vi "Lift.vi"   [LabVIEW 2017]
uses:
  <userlib>/836-Library/System/QCP_V2/QCPSupportCode/QCPData.ctl
  <userlib>/836-Library/System/QCP_V2/QCPSupportCode/QCP_GetDbl.vi
types:
  T1 = typedef "Semaphore RefNum" = refnum<k1>
  T2 = cluster{"Data Value Refnum":refnum<data-value>, "semaphore":T1}
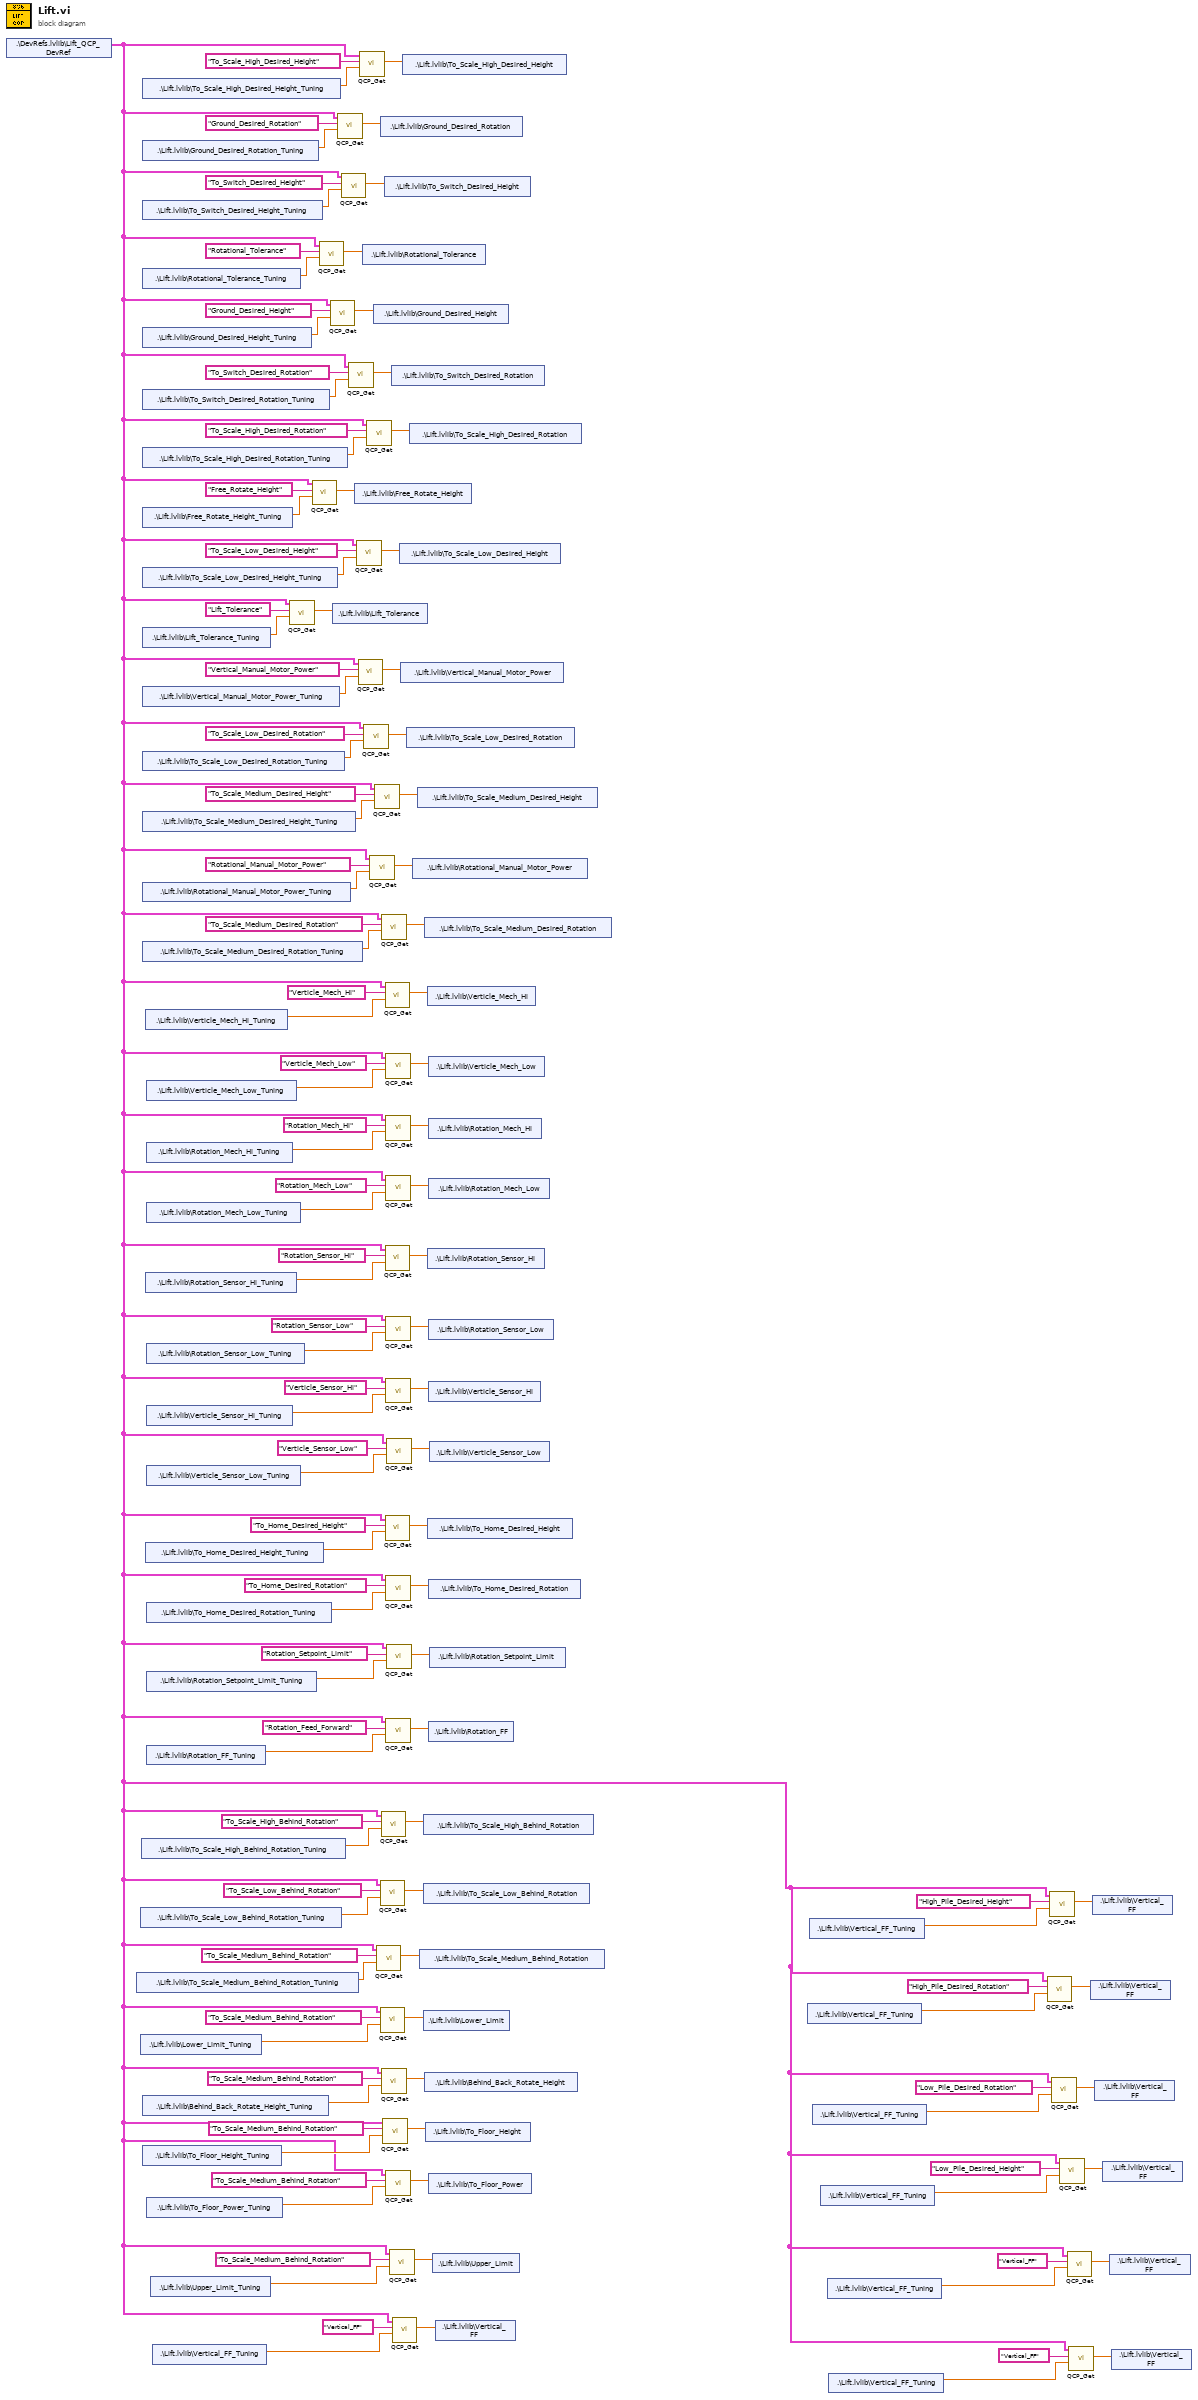
[diagram p0: block diagram]
diagram:
  n1 = shared-variable ".\\DevRefs.lvlib\\Lift_QCP_DevRef"() -> (w1:T2)  [unwired: 1 in, 1 out]
  n2 = shared-variable ".\\Lift.lvlib\\To_Scale_Medium_Behind_Rotation_Tuninig"() -> (w38:dbl)  [unwired: 1 in, 1 out]
  n3 = shared-variable ".\\Lift.lvlib\\To_Scale_Low_Behind_Rotation_Tuning"() -> (w43:dbl)  [unwired: 1 in, 1 out]
  n4 = shared-variable ".\\Lift.lvlib\\Lower_Limit_Tuning"() -> (w37:dbl)  [unwired: 1 in, 1 out]
  n5 = shared-variable ".\\Lift.lvlib\\To_Scale_High_Behind_Rotation_Tuning"() -> (w44:dbl)  [unwired: 1 in, 1 out]
  n6 = shared-variable ".\\Lift.lvlib\\To_Scale_High_Desired_Height_Tuning"() -> (w91:dbl)  [unwired: 1 in, 1 out]
  n7 = shared-variable ".\\Lift.lvlib\\Ground_Desired_Rotation_Tuning"() -> (w95:dbl)  [unwired: 1 in, 1 out]
  n8 = shared-variable ".\\Lift.lvlib\\To_Switch_Desired_Height_Tuning"() -> (w85:dbl)  [unwired: 1 in, 1 out]
  n9 = shared-variable ".\\Lift.lvlib\\Rotational_Tolerance_Tuning"() -> (w92:dbl)  [unwired: 1 in, 1 out]
  n10 = shared-variable ".\\Lift.lvlib\\Ground_Desired_Height_Tuning"() -> (w96:dbl)  [unwired: 1 in, 1 out]
  n11 = shared-variable ".\\Lift.lvlib\\To_Switch_Desired_Rotation_Tuning"() -> (w84:dbl)  [unwired: 1 in, 1 out]
  n12 = shared-variable ".\\Lift.lvlib\\To_Scale_High_Desired_Rotation_Tuning"() -> (w90:dbl)  [unwired: 1 in, 1 out]
  n13 = shared-variable ".\\Lift.lvlib\\Free_Rotate_Height_Tuning"() -> (w97:dbl)  [unwired: 1 in, 1 out]
  n14 = shared-variable ".\\Lift.lvlib\\To_Scale_Low_Desired_Height_Tuning"() -> (w89:dbl)  [unwired: 1 in, 1 out]
  n15 = shared-variable ".\\Lift.lvlib\\Lift_Tolerance_Tuning"() -> (w94:dbl)  [unwired: 1 in, 1 out]
  n16 = shared-variable ".\\Lift.lvlib\\Vertical_Manual_Motor_Power_Tuning"() -> (w83:dbl)  [unwired: 1 in, 1 out]
  n17 = shared-variable ".\\Lift.lvlib\\To_Scale_Low_Desired_Rotation_Tuning"() -> (w88:dbl)  [unwired: 1 in, 1 out]
  n18 = shared-variable ".\\Lift.lvlib\\To_Scale_Medium_Desired_Height_Tuning"() -> (w87:dbl)  [unwired: 1 in, 1 out]
  n19 = shared-variable ".\\Lift.lvlib\\Rotational_Manual_Motor_Power_Tuning"() -> (w93:dbl)  [unwired: 1 in, 1 out]
  n20 = shared-variable ".\\Lift.lvlib\\To_Scale_Medium_Desired_Rotation_Tuning"() -> (w86:dbl)  [unwired: 1 in, 1 out]
  n21 = shared-variable ".\\Lift.lvlib\\Behind_Back_Rotate_Height_Tuning"() -> (w32:dbl)  [unwired: 1 in, 1 out]
  n22 = shared-variable ".\\Lift.lvlib\\To_Floor_Height_Tuning"() -> (w31:dbl)  [unwired: 1 in, 1 out]
  n23 = shared-variable ".\\Lift.lvlib\\Verticle_Mech_Hi_Tuning"() -> (w82:dbl)  [unwired: 1 in, 1 out]
  n24 = shared-variable ".\\Lift.lvlib\\Rotation_Sensor_Hi_Tuning"() -> (w59:dbl)  [unwired: 1 in, 1 out]
  n25 = shared-variable ".\\Lift.lvlib\\To_Home_Desired_Height_Tuning"() -> (w58:dbl)  [unwired: 1 in, 1 out]
  n26 = shared-variable ".\\Lift.lvlib\\Verticle_Mech_Low_Tuning"() -> (w77:dbl)  [unwired: 1 in, 1 out]
  n27 = shared-variable ".\\Lift.lvlib\\Rotation_Mech_Hi_Tuning"() -> (w76:dbl)  [unwired: 1 in, 1 out]
  n28 = shared-variable ".\\Lift.lvlib\\Rotation_Mech_Low_Tuning"() -> (w71:dbl)  [unwired: 1 in, 1 out]
  n29 = shared-variable ".\\Lift.lvlib\\Rotation_Sensor_Low_Tuning"() -> (w64:dbl)  [unwired: 1 in, 1 out]
  n30 = shared-variable ".\\Lift.lvlib\\Verticle_Sensor_Hi_Tuning"() -> (w65:dbl)  [unwired: 1 in, 1 out]
  n31 = shared-variable ".\\Lift.lvlib\\To_Home_Desired_Rotation_Tuning"() -> (w53:dbl)  [unwired: 1 in, 1 out]
  n32 = shared-variable ".\\Lift.lvlib\\Rotation_FF_Tuning"() -> (w49:dbl)  [unwired: 1 in, 1 out]
  n33 = shared-variable ".\\Lift.lvlib\\To_Floor_Power_Tuning"() -> (w26:dbl)  [unwired: 1 in, 1 out]
  n34 = shared-variable ".\\Lift.lvlib\\Verticle_Sensor_Low_Tuning"() -> (w70:dbl)  [unwired: 1 in, 1 out]
  n35 = shared-variable ".\\Lift.lvlib\\Rotation_Setpoint_Limit_Tuning"() -> (w50:dbl)  [unwired: 1 in, 1 out]
  n36 = shared-variable ".\\Lift.lvlib\\Upper_Limit_Tuning"() -> (w25:dbl)  [unwired: 1 in, 1 out]
  n37 = shared-variable ".\\Lift.lvlib\\Vertical_FF_Tuning"() -> (w20:dbl)  [unwired: 1 in, 1 out]
  n38 = call-poly <userlib>:"QCP_Get.vi"("Tuning Value"=w94, "Value Name"="Lift_Tolerance", "QCP_DevRef_In"=w1) -> ("Value"=w109:dbl)  [unwired: 6 in, 2 out]
  n39 = call-poly <userlib>:"QCP_Get.vi"("Tuning Value"=w97, "Value Name"="Free_Rotate_Height", "QCP_DevRef_In"=w1) -> ("Value"=w112:dbl)  [unwired: 6 in, 2 out]
  n40 = call-poly <userlib>:"QCP_Get.vi"("Tuning Value"=w92, "Value Name"="Rotational_Tolerance", "QCP_DevRef_In"=w1) -> ("Value"=w104:dbl)  [unwired: 6 in, 2 out]
  n41 = call-poly <userlib>:"QCP_Get.vi"("Tuning Value"=w96, "Value Name"="Ground_Desired_Height", "QCP_DevRef_In"=w1) -> ("Value"=w111:dbl)  [unwired: 6 in, 2 out]
  n42 = shared-variable ".\\Lift.lvlib\\Lift_Tolerance"(w109) -> ()  [unwired: 1 in, 1 out]
  n43 = call-poly <userlib>:"QCP_Get.vi"("Tuning Value"=w95, "Value Name"="Ground_Desired_Rotation", "QCP_DevRef_In"=w1) -> ("Value"=w110:dbl)  [unwired: 6 in, 2 out]
  n44 = call-poly <userlib>:"QCP_Get.vi"("Tuning Value"=w85, "Value Name"="To_Switch_Desired_Height", "QCP_DevRef_In"=w1) -> ("Value"=w100:dbl)  [unwired: 6 in, 2 out]
  n45 = call-poly <userlib>:"QCP_Get.vi"("Tuning Value"=w84, "Value Name"="To_Switch_Desired_Rotation", "QCP_DevRef_In"=w1) -> ("Value"=w99:dbl)  [unwired: 6 in, 2 out]
  n46 = shared-variable ".\\Lift.lvlib\\Free_Rotate_Height"(w112) -> ()  [unwired: 1 in, 1 out]
  n47 = call-poly <userlib>:"QCP_Get.vi"("Tuning Value"=w89, "Value Name"="To_Scale_Low_Desired_Height", "QCP_DevRef_In"=w1) -> ("Value"=w105:dbl)  [unwired: 6 in, 2 out]
  n48 = call-poly <userlib>:"QCP_Get.vi"("Tuning Value"=w83, "Value Name"="Vertical_Manual_Motor_Power", "QCP_DevRef_In"=w1) -> ("Value"=w98:dbl)  [unwired: 6 in, 2 out]
  n49 = call-poly <userlib>:"QCP_Get.vi"("Tuning Value"=w91, "Value Name"="To_Scale_High_Desired_Height", "QCP_DevRef_In"=w1) -> ("Value"=w107:dbl)  [unwired: 6 in, 2 out]
  n50 = shared-variable ".\\Lift.lvlib\\Rotational_Tolerance"(w104) -> ()  [unwired: 1 in, 1 out]
  n51 = call-poly <userlib>:"QCP_Get.vi"("Tuning Value"=w88, "Value Name"="To_Scale_Low_Desired_Rotation", "QCP_DevRef_In"=w1) -> ("Value"=w102:dbl)  [unwired: 6 in, 2 out]
  n52 = call-poly <userlib>:"QCP_Get.vi"("Tuning Value"=w90, "Value Name"="To_Scale_High_Desired_Rotation", "QCP_DevRef_In"=w1) -> ("Value"=w103:dbl)  [unwired: 6 in, 2 out]
  n53 = call-poly <userlib>:"QCP_Get.vi"("Tuning Value"=w93, "Value Name"="Rotational_Manual_Motor_Power", "QCP_DevRef_In"=w1) -> ("Value"=w108:dbl)  [unwired: 6 in, 2 out]
  n54 = shared-variable ".\\Lift.lvlib\\Ground_Desired_Height"(w111) -> ()  [unwired: 1 in, 1 out]
  n55 = call-poly <userlib>:"QCP_Get.vi"("Tuning Value"=w87, "Value Name"="To_Scale_Medium_Desired_Height", "QCP_DevRef_In"=w1) -> ("Value"=w101:dbl)  [unwired: 6 in, 2 out]
  n56 = call-poly <userlib>:"QCP_Get.vi"("Tuning Value"=w38, "Value Name"="To_Scale_Medium_Behind_Rotation", "QCP_DevRef_In"=w1) -> ("Value"=w39:dbl)  [unwired: 6 in, 2 out]
  n57 = shared-variable ".\\Lift.lvlib\\Ground_Desired_Rotation"(w110) -> ()  [unwired: 1 in, 1 out]
  n58 = call-poly <userlib>:"QCP_Get.vi"("Tuning Value"=w43, "Value Name"="To_Scale_Low_Behind_Rotation", "QCP_DevRef_In"=w1) -> ("Value"=w42:dbl)  [unwired: 6 in, 2 out]
  n59 = call-poly <userlib>:"QCP_Get.vi"("Tuning Value"=w37, "Value Name"="To_Scale_Medium_Behind_Rotation", "QCP_DevRef_In"=w1) -> ("Value"=w36:dbl)  [unwired: 6 in, 2 out]
  n60 = call-poly <userlib>:"QCP_Get.vi"("Tuning Value"=w44, "Value Name"="To_Scale_High_Behind_Rotation", "QCP_DevRef_In"=w1) -> ("Value"=w45:dbl)  [unwired: 6 in, 2 out]
  n61 = call-poly <userlib>:"QCP_Get.vi"("Tuning Value"=w86, "Value Name"="To_Scale_Medium_Desired_Rotation", "QCP_DevRef_In"=w1) -> ("Value"=w106:dbl)  [unwired: 6 in, 2 out]
  n62 = call-poly <userlib>:"QCP_Get.vi"("Tuning Value"=w32, "Value Name"="To_Scale_Medium_Behind_Rotation", "QCP_DevRef_In"=w1) -> ("Value"=w33:dbl)  [unwired: 6 in, 2 out]
  n63 = call-poly <userlib>:"QCP_Get.vi"("Tuning Value"=w31, "Value Name"="To_Scale_Medium_Behind_Rotation", "QCP_DevRef_In"=w1) -> ("Value"=w30:dbl)  [unwired: 6 in, 2 out]
  n64 = shared-variable ".\\Lift.lvlib\\To_Switch_Desired_Height"(w100) -> ()  [unwired: 1 in, 1 out]
  n65 = call-poly <userlib>:"QCP_Get.vi"("Tuning Value"=w82, "Value Name"="Verticle_Mech_Hi", "QCP_DevRef_In"=w1) -> ("Value"=w81:dbl)  [unwired: 6 in, 2 out]
  n66 = call-poly <userlib>:"QCP_Get.vi"("Tuning Value"=w59, "Value Name"="Rotation_Sensor_Hi", "QCP_DevRef_In"=w1) -> ("Value"=w60:dbl)  [unwired: 6 in, 2 out]
  n67 = call-poly <userlib>:"QCP_Get.vi"("Tuning Value"=w58, "Value Name"="To_Home_Desired_Height", "QCP_DevRef_In"=w1) -> ("Value"=w57:dbl)  [unwired: 6 in, 2 out]
  n68 = call-poly <userlib>:"QCP_Get.vi"("Tuning Value"=w77, "Value Name"="Verticle_Mech_Low", "QCP_DevRef_In"=w1) -> ("Value"=w78:dbl)  [unwired: 6 in, 2 out]
  n69 = call-poly <userlib>:"QCP_Get.vi"("Tuning Value"=w76, "Value Name"="Rotation_Mech_Hi", "QCP_DevRef_In"=w1) -> ("Value"=w75:dbl)  [unwired: 6 in, 2 out]
  n70 = call-poly <userlib>:"QCP_Get.vi"("Tuning Value"=w71, "Value Name"="Rotation_Mech_Low", "QCP_DevRef_In"=w1) -> ("Value"=w72:dbl)  [unwired: 6 in, 2 out]
  n71 = call-poly <userlib>:"QCP_Get.vi"("Tuning Value"=w64, "Value Name"="Rotation_Sensor_Low", "QCP_DevRef_In"=w1) -> ("Value"=w63:dbl)  [unwired: 6 in, 2 out]
  n72 = call-poly <userlib>:"QCP_Get.vi"("Tuning Value"=w65, "Value Name"="Verticle_Sensor_Hi", "QCP_DevRef_In"=w1) -> ("Value"=w66:dbl)  [unwired: 6 in, 2 out]
  n73 = call-poly <userlib>:"QCP_Get.vi"("Tuning Value"=w53, "Value Name"="To_Home_Desired_Rotation", "QCP_DevRef_In"=w1) -> ("Value"=w54:dbl)  [unwired: 6 in, 2 out]
  n74 = call-poly <userlib>:"QCP_Get.vi"("Tuning Value"=w49, "Value Name"="Rotation_Feed_Forward", "QCP_DevRef_In"=w1) -> ("Value"=w48:dbl)  [unwired: 6 in, 2 out]
  n75 = call-poly <userlib>:"QCP_Get.vi"("Tuning Value"=w26, "Value Name"="To_Scale_Medium_Behind_Rotation", "QCP_DevRef_In"=w1) -> ("Value"=w27:dbl)  [unwired: 6 in, 2 out]
  n76 = call-poly <userlib>:"QCP_Get.vi"("Tuning Value"=w70, "Value Name"="Verticle_Sensor_Low", "QCP_DevRef_In"=w1) -> ("Value"=w69:dbl)  [unwired: 6 in, 2 out]
  n77 = call-poly <userlib>:"QCP_Get.vi"("Tuning Value"=w50, "Value Name"="Rotation_Setpoint_Limit", "QCP_DevRef_In"=w1) -> ("Value"=w51:dbl)  [unwired: 6 in, 2 out]
  n78 = call-poly <userlib>:"QCP_Get.vi"("Tuning Value"=w25, "Value Name"="To_Scale_Medium_Behind_Rotation", "QCP_DevRef_In"=w1) -> ("Value"=w24:dbl)  [unwired: 6 in, 2 out]
  n79 = shared-variable ".\\Lift.lvlib\\To_Switch_Desired_Rotation"(w99) -> ()  [unwired: 1 in, 1 out]
  n80 = call-poly <userlib>:"QCP_Get.vi"("Tuning Value"=w20, "Value Name"="Vertical_FF", "QCP_DevRef_In"=w1) -> ("Value"=w21:dbl)  [unwired: 6 in, 2 out]
  n81 = shared-variable ".\\Lift.lvlib\\To_Scale_Low_Desired_Height"(w105) -> ()  [unwired: 1 in, 1 out]
  n82 = shared-variable ".\\Lift.lvlib\\Vertical_Manual_Motor_Power"(w98) -> ()  [unwired: 1 in, 1 out]
  n83 = shared-variable ".\\Lift.lvlib\\To_Scale_High_Desired_Height"(w107) -> ()  [unwired: 1 in, 1 out]
  n84 = shared-variable ".\\Lift.lvlib\\To_Scale_Low_Desired_Rotation"(w102) -> ()  [unwired: 1 in, 1 out]
  n85 = shared-variable ".\\Lift.lvlib\\To_Scale_High_Desired_Rotation"(w103) -> ()  [unwired: 1 in, 1 out]
  n86 = shared-variable ".\\Lift.lvlib\\Rotational_Manual_Motor_Power"(w108) -> ()  [unwired: 1 in, 1 out]
  n87 = shared-variable ".\\Lift.lvlib\\To_Scale_Medium_Desired_Height"(w101) -> ()  [unwired: 1 in, 1 out]
  n88 = shared-variable ".\\Lift.lvlib\\To_Scale_Medium_Behind_Rotation"(w39) -> ()  [unwired: 1 in, 1 out]
  n89 = shared-variable ".\\Lift.lvlib\\To_Scale_Low_Behind_Rotation"(w42) -> ()  [unwired: 1 in, 1 out]
  n90 = shared-variable ".\\Lift.lvlib\\Lower_Limit"(w36) -> ()  [unwired: 1 in, 1 out]
  n91 = shared-variable ".\\Lift.lvlib\\To_Scale_High_Behind_Rotation"(w45) -> ()  [unwired: 1 in, 1 out]
  n92 = shared-variable ".\\Lift.lvlib\\To_Scale_Medium_Desired_Rotation"(w106) -> ()  [unwired: 1 in, 1 out]
  n93 = shared-variable ".\\Lift.lvlib\\Behind_Back_Rotate_Height"(w33) -> ()  [unwired: 1 in, 1 out]
  n94 = shared-variable ".\\Lift.lvlib\\To_Floor_Height"(w30) -> ()  [unwired: 1 in, 1 out]
  n95 = shared-variable ".\\Lift.lvlib\\Verticle_Mech_Hi"(w81) -> ()  [unwired: 1 in, 1 out]
  n96 = shared-variable ".\\Lift.lvlib\\Rotation_Sensor_Hi"(w60) -> ()  [unwired: 1 in, 1 out]
  n97 = shared-variable ".\\Lift.lvlib\\To_Home_Desired_Height"(w57) -> ()  [unwired: 1 in, 1 out]
  n98 = shared-variable ".\\Lift.lvlib\\Verticle_Mech_Low"(w78) -> ()  [unwired: 1 in, 1 out]
  n99 = shared-variable ".\\Lift.lvlib\\Rotation_Mech_Hi"(w75) -> ()  [unwired: 1 in, 1 out]
  n100 = shared-variable ".\\Lift.lvlib\\Rotation_Mech_Low"(w72) -> ()  [unwired: 1 in, 1 out]
  n101 = shared-variable ".\\Lift.lvlib\\Rotation_Sensor_Low"(w63) -> ()  [unwired: 1 in, 1 out]
  n102 = shared-variable ".\\Lift.lvlib\\Verticle_Sensor_Hi"(w66) -> ()  [unwired: 1 in, 1 out]
  n103 = shared-variable ".\\Lift.lvlib\\To_Home_Desired_Rotation"(w54) -> ()  [unwired: 1 in, 1 out]
  n104 = shared-variable ".\\Lift.lvlib\\Rotation_FF"(w48) -> ()  [unwired: 1 in, 1 out]
  n105 = shared-variable ".\\Lift.lvlib\\To_Floor_Power"(w27) -> ()  [unwired: 1 in, 1 out]
  n106 = shared-variable ".\\Lift.lvlib\\Verticle_Sensor_Low"(w69) -> ()  [unwired: 1 in, 1 out]
  n107 = shared-variable ".\\Lift.lvlib\\Rotation_Setpoint_Limit"(w51) -> ()  [unwired: 1 in, 1 out]
  n108 = shared-variable ".\\Lift.lvlib\\Upper_Limit"(w24) -> ()  [unwired: 1 in, 1 out]
  n109 = shared-variable ".\\Lift.lvlib\\Vertical_FF"(w21) -> ()  [unwired: 1 in, 1 out]
  n110 = shared-variable ".\\Lift.lvlib\\Vertical_FF_Tuning"() -> (w14:dbl)  [unwired: 1 in, 1 out]
  n111 = shared-variable ".\\Lift.lvlib\\Vertical_FF_Tuning"() -> (w17:dbl)  [unwired: 1 in, 1 out]
  n112 = shared-variable ".\\Lift.lvlib\\Vertical_FF_Tuning"() -> (w11:dbl)  [unwired: 1 in, 1 out]
  n113 = shared-variable ".\\Lift.lvlib\\Vertical_FF_Tuning"() -> (w8:dbl)  [unwired: 1 in, 1 out]
  n114 = shared-variable ".\\Lift.lvlib\\Vertical_FF_Tuning"() -> (w5:dbl)  [unwired: 1 in, 1 out]
  n115 = shared-variable ".\\Lift.lvlib\\Vertical_FF_Tuning"() -> (w2:dbl)  [unwired: 1 in, 1 out]
  n116 = call-poly <userlib>:"QCP_Get.vi"("Tuning Value"=w14, "Value Name"="High_Pile_Desired_Rotation", "QCP_DevRef_In"=w1) -> ("Value"=w15:dbl)  [unwired: 6 in, 2 out]
  n117 = call-poly <userlib>:"QCP_Get.vi"("Tuning Value"=w17, "Value Name"="High_Pile_Desired_Height", "QCP_DevRef_In"=w1) -> ("Value"=w18:dbl)  [unwired: 6 in, 2 out]
  n118 = call-poly <userlib>:"QCP_Get.vi"("Tuning Value"=w11, "Value Name"="Low_Pile_Desired_Rotation", "QCP_DevRef_In"=w1) -> ("Value"=w12:dbl)  [unwired: 6 in, 2 out]
  n119 = call-poly <userlib>:"QCP_Get.vi"("Tuning Value"=w8, "Value Name"="Low_Pile_Desired_Height", "QCP_DevRef_In"=w1) -> ("Value"=w9:dbl)  [unwired: 6 in, 2 out]
  n120 = call-poly <userlib>:"QCP_Get.vi"("Tuning Value"=w5, "Value Name"="Vertical_FF", "QCP_DevRef_In"=w1) -> ("Value"=w6:dbl)  [unwired: 6 in, 2 out]
  n121 = call-poly <userlib>:"QCP_Get.vi"("Tuning Value"=w2, "Value Name"="Vertical_FF", "QCP_DevRef_In"=w1) -> ("Value"=w3:dbl)  [unwired: 6 in, 2 out]
  n122 = shared-variable ".\\Lift.lvlib\\Vertical_FF"(w15) -> ()  [unwired: 1 in, 1 out]
  n123 = shared-variable ".\\Lift.lvlib\\Vertical_FF"(w18) -> ()  [unwired: 1 in, 1 out]
  n124 = shared-variable ".\\Lift.lvlib\\Vertical_FF"(w12) -> ()  [unwired: 1 in, 1 out]
  n125 = shared-variable ".\\Lift.lvlib\\Vertical_FF"(w9) -> ()  [unwired: 1 in, 1 out]
  n126 = shared-variable ".\\Lift.lvlib\\Vertical_FF"(w6) -> ()  [unwired: 1 in, 1 out]
  n127 = shared-variable ".\\Lift.lvlib\\Vertical_FF"(w3) -> ()  [unwired: 1 in, 1 out]
